vi "Subtract.vi"   [LabVIEW 2020, in "NI_Matrix.lvlib"]
doc: "Computes the difference of the inputs."
uses:
  <vilib>/Analysis/Matrix/NI_Matrix.lvlib
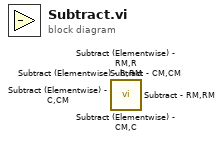
[diagram p0: block diagram]
diagram:
  n1 = call <vilib>:"Subtract (Elementwise) - CM,C.vi"() -> ()  [unwired: 2 in, 1 out]
  n2 = call <vilib>:"Subtract - CM,CM.vi"() -> ()  [unwired: 2 in, 1 out]
  n3 = call <vilib>:"Subtract (Elementwise) - C,CM.vi"() -> ()  [unwired: 2 in, 1 out]
  n4 = call <vilib>:"Subtract - RM,RM.vi"() -> ()  [unwired: 2 in, 1 out]
  n5 = call <vilib>:"Subtract (Elementwise) - RM,R.vi"() -> ()  [unwired: 2 in, 1 out]
  n6 = call <vilib>:"Subtract (Elementwise) - R,RM.vi"() -> ()  [unwired: 2 in, 1 out]
